vi "Update Parameters Configuration File Error.vi"(8 "error in":errorcluster, 11 "configuration files ref in":T1 format="%.0x") -> (0 "error out":errorcluster, 3 "configuration files ref out":T1 format="%.0x")   [LabVIEW 2020, in "AIM MIL-STD-1553 Scripting.lvlib"]
uses:
  AIM MIL-STD-1553 Scripting.lvlib
  <vilib>/NI VeriStand/Custom Device API/Custom Device API.lvlib
  Constants.vi
  <vilib>/NI VeriStand/Custom Device API/Custom Device Item Ref.ctl
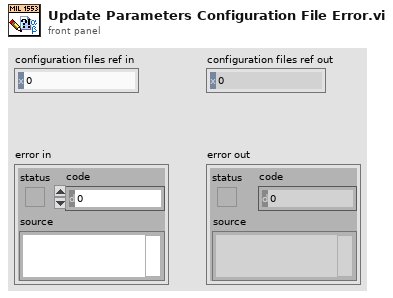
[diagram p1: front panel]
types:
  T1 = typedef "Custom Device API.lvlib/Custom Device Item Ref.ctl" = u64
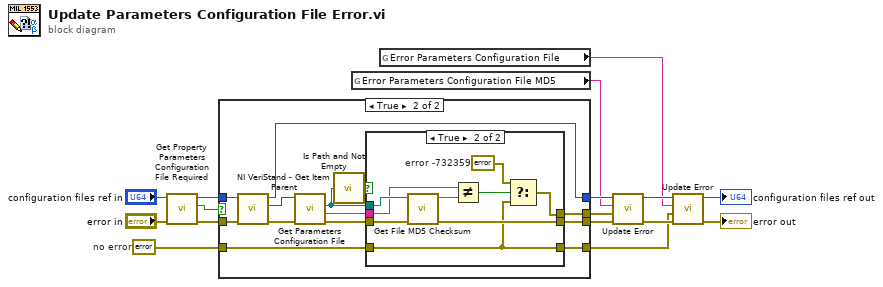
[diagram p0: block diagram]
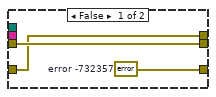
[diagram p3: hidden frame]
diagram:
  w11 = errorcluster {"status"=FALSE, "code"=0, "source"=""}  # no error
  n1 = call "Get Property Parameters Configuration File Required.vi"("error in"="error in", "configuration files ref"="configuration files ref in") -> ("error out"=w13:errorcluster, "required"=w14:bool, "configuration files ref out"=w12:T1)  [unwired: 6 in, 1 out]
  n2 = case shown="True" w14 {
    tunnel: w13 -> [w19 w32]
    tunnel: [w19 w23] -> w7
    tunnel: w12 -> [w18 w31]
    tunnel: [w18 w24] -> w8
    tunnel: w11 -> [w17 w22]
    tunnel: [w17 w21] -> w4
    tunnel: [w17 w20] -> w3
    frame False {
    }
    frame True {
      n3 = call <vilib>:"NI VeriStand - Get Item Parent.vi"("error in (no error)"=w32, "Item Ref in"=w31) -> ("error out"=w30:errorcluster, "Parent Ref"=w29:T1, "Item Ref out"=w24:T1)  [unwired: 6 in, 1 out]
      n4 = call "Get Parameters Configuration File.vi"("error in"=w30, "Ballard MIL-STD 1553 custom device in"=w29) -> ("error out"=w26:errorcluster, "MD5 checksum"=w28:string, "parameters configuration file"=w27:path)  [unwired: 6 in, 1 out]
      n5 = call <vilib>:"Is Path and Not Empty.vi"("path"=w27) -> ("Is Path and Not Empty?"=w25:bool)  [unwired: 4 in]
      n6 = case shown="True" w25 {
        tunnel: w28 -> [_ w40]
        tunnel: w27 -> [_ w43]
        tunnel: w26 -> [w35 w44]
        tunnel: [w35 w42] -> w23
        tunnel: [w33 w37] -> w21
        tunnel: w22 -> [w33 w36]
        tunnel: [w34 w36] -> w20
        frame False {
          w34 = errorcluster {"status"=TRUE, "code"=-732357, "source"="parameters configuration file path must not be empty."}  # error -732357
        }
        frame True {
          w38 = errorcluster {"status"=TRUE, "code"=-732359, "source"="parameters configuration file changed since import."}  # error -732359
          n7 = call "Get File MD5 Checksum.vi"("error in"=w44, "path"=w43) -> ("error out"=w42:errorcluster, "MD5"=w41:string)  [unwired: 8 in]
          n8 = Not Equal?(x=w40, y=w41) -> (x != y?=w39:bool)
          n9 = Select(t=w38, s=w39, f=w36) -> (s? t:f=w37:errorcluster)
        }
      }
    }
  }
  n10 = global read "Constants.vi" "Error Parameters Configuration File MD5"() -> (w1:string)
  n11 = global read "Constants.vi" "Error Parameters Configuration File"() -> (w2:string)
  n12 = call "Update Error.vi"("error in"=w7, "error to report"=w4, "error key"=w1, "section ref in"=w8) -> ("error out"=w9:errorcluster, "section ref out"=w10:T1)  [unwired: 6 in]
  n13 = call "Update Error.vi"("error in"=w9, "error to report"=w3, "error key"=w2, "section ref in"=w10) -> ("error out"=→"error out":errorcluster, "section ref out"=→"configuration files ref out":T1)  [unwired: 6 in]
